vi "dataTypesExample.vi"() -> ()   [LabVIEW 2014]
panel:
  out "Converted Floating Point Indicator":dbl
  out "1D Floating Point Array Indicator":dbl[](array[numeric])
  out "Coerced Floating Point Indicator":dbl
  out "Integer Indicator":i16
  out "String Indicator":string
  out "Floating Point Indicator":dbl
  in  "1D Floating Point Array":dbl[](array[numeric])
  in  "String":string
  in  "Integer":i16
  in  "Floating Point":dbl
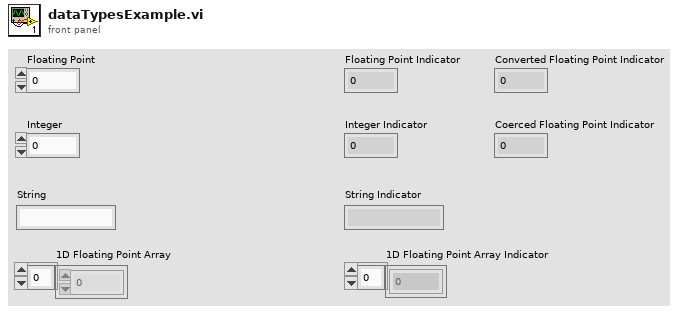
[diagram p1: front panel]
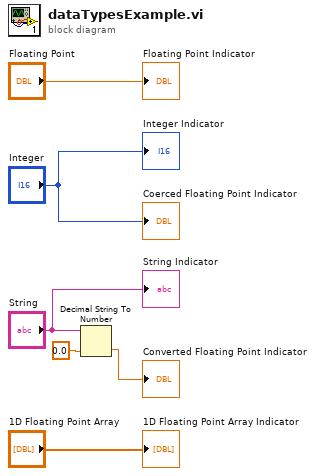
[diagram p0: block diagram]
diagram:
  n1 = Decimal String To Number(string="String", default (0L)=0.0 ("default (0 I32)")) -> (number=→"Converted Floating Point Indicator":dbl)  [unwired: 1 in, 1 out]
  "Floating Point Indicator" <- "Floating Point"
  "String Indicator" <- "String"
  "Integer Indicator" <- "Integer"
  "Coerced Floating Point Indicator" <- "Integer"
  "1D Floating Point Array Indicator" <- "1D Floating Point Array"
